vi "Execute Build Target.vi"(7 "LabVIEW Previous Version":T1=enum."2015", 8 "Error In":errorcluster, 11 "Target Project Root In":path) -> (0 "Error Out":errorcluster, 3 "Target Project Root Out":path)   [LabVIEW 2017]
doc: "Executes building a project/target using the System Exec.vi to start a specific version of LabVIEW with the \"Build Target.vi\" as an argument. Since the \"Build Target.vi\" is configured to run when loaded, this will immediate build all of the components and the VI package from within the specific version of LabVIEW.\n\nThe VI Server cannot be used here. The System Exec.vi must be used to ensure the correct version of LabVIEW is used to open and run the \"Build Target.vi\". The VI Server will use the LabVIEW environment that is executing this VI, not the correct version."
uses:
  LabVIEW Versions.ctl
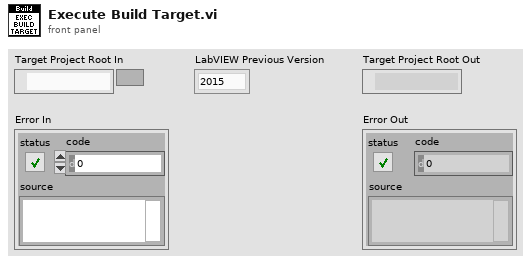
[diagram p1: front panel]
types:
  T1 = typedef "LabVIEW Versions.ctl" = enum16{"2009", "2010", "2011", "2012", "2013", "2014", "2015", "2016", "2017", "2018"}
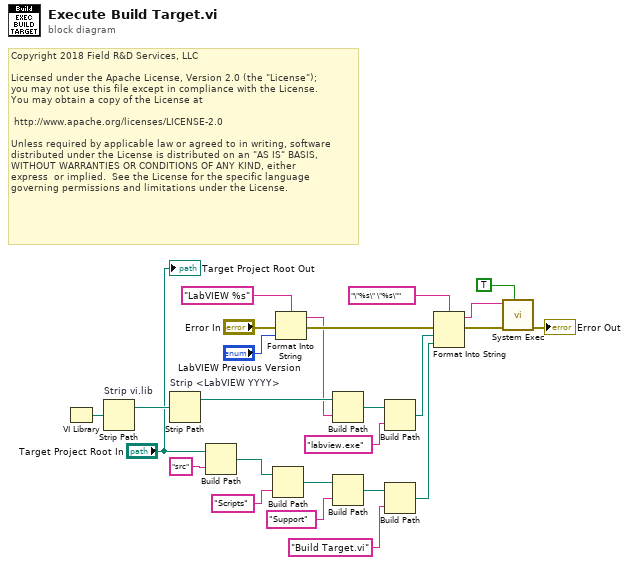
[diagram p0: block diagram]
diagram:
  # "Copyright 2018 Field R&D Services, LLC\n\nLicensed under the Apache License, Version 2.0 (the \"License\");\nyou may not use this file except in compliance with the License.\nYou may obtain a copy of the License at\n\n\thttp://www.apache.org/licenses/LICENSE-2.0\n\nUnless required by applicable law or agreed to in writing, software\ndistributed under the License is distributed on an \"AS IS\" BASIS,\nWITHOUT WARRANTIES OR CONDITIONS OF ANY KIND, either \nexpress  or implied.  See the License for the specific language \ngoverning permissions and limitations under the License."
  n1 = VI Library() -> (path=w24:path)
  n2 = Strip Path "Strip vi.lib"(path=w24) -> (stripped path=w23:path)  [unwired: 1 out]
  n3 = Strip Path "Strip <LabVIEW YYYY>"(path=w23) -> (stripped path=w22:path)  [unwired: 1 out]
  n4 = Build Path(base path="Target Project Root In", name or relative path="src") -> (appended path=w7:path)
  n5 = Build Path(base path=w7, name or relative path="Scripts") -> (appended path=w5:path)
  n6 = Format Into String(format string="LabVIEW %s", error in="Error In", "LabVIEW Previous Version") -> (resulting string=w19:string, error out=w21:errorcluster)  [unwired: 1 in]
  n7 = Build Path(base path=w22, name or relative path=w19) -> (appended path=w18:path)
  n8 = Build Path(base path=w5, name or relative path="Support") -> (appended path=w3:path)
  n9 = Build Path(base path=w18, name or relative path="labview.exe") -> (appended path=w11:path)
  n10 = Build Path(base path=w3, name or relative path="Build Target.vi") -> (appended path=w15:path)
  n11 = Format Into String(format string="\"%s\" \"%s\"", error in=w21, w11, w15) -> (resulting string=w10:string, error out=w13:errorcluster)  [unwired: 1 in]
  n12 = call <vilib>:"System Exec.vi"("wait until completion? (T)"=TRUE, "error in (no error)"=w13, "command line"=w10) -> ("error out"=→"Error Out":errorcluster)  [unwired: 5 in, 3 out]
  "Target Project Root Out" <- "Target Project Root In"
